vi "Get Request Type.vi"(8 "error in (no error)":errorcluster, 11 "GetInputDefaultSettings in":refnum<class "GetInputDefaultSettings.lvclass">) -> (0 "error out":errorcluster, 2 "Request Type":string, 3 "GetInputDefaultSettings out":refnum<class "GetInputDefaultSettings.lvclass">)   [LabVIEW 2020, in "obs-websocket.lvlib" / "GetInputDefaultSettings.lvclass"]
uses:
  GetInputDefaultSettings.lvclass
  GetInputDefaultSettings.lvclass/GetInputDefaultSettings.ctl
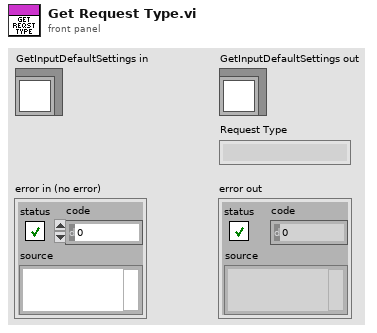
[diagram p1: front panel]
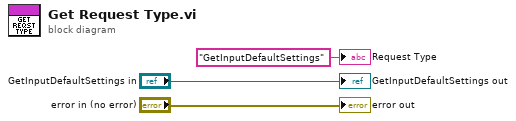
[diagram p0: block diagram]
diagram:
  "error out" <- "error in (no error)"
  "GetInputDefaultSettings out" <- "GetInputDefaultSettings in"
  "Request Type" <- "GetInputDefaultSettings" ("Request Type")
